vi "FourCC String to Int.vi"(10 "error in (no error)":errorcluster, 11 "fourCC String":string="MJPG") -> (2 "error out":errorcluster, 3 "fourCC Int":i32)   [LabVIEW 2014]
doc: "Help VI to convert the FourCC String to Int and back"
uses:
  Dependencies/x86/MSC I Process32.dll
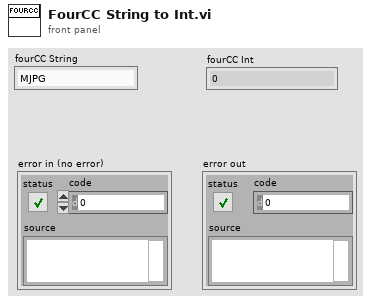
[diagram p1: front panel]
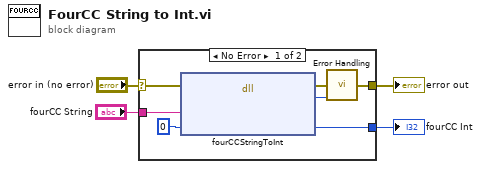
[diagram p0: block diagram]
diagram:
  n1 = case shown="No Error" "error in (no error)" {
    selector: "error in (no error)" -> [w9 w12]
    tunnel: [w8 w12] -> w4
    tunnel: "fourCC String" -> [w5 _]
    tunnel: [w6 _] -> w1
    frame No Error {
      n2 = dll-call lib="C:/Users/MSC/LabVIEW Projekte/LV 2014/MSC I-Process/user.lib/MSC-I Process/Dependencies/x86/MSC I Process*.dll" fn="fourCCStringToInt"(error in=w9, "fourCCString"=w5, "fourCCInt"=0) -> (error out=w11:errorcluster, "error"=w10:i32, "fourCCInt"=w6:i32)  [unwired: 3 in, 1 out]
      n3 = call "Error Handling.vi"("error in (no error)"=w11, "return type"=w10) -> ("error out"=w8:errorcluster)  [unwired: 12 in, 1 out]
    }
    frame Error {
    }
  }
  "error out" <- w4
  "fourCC Int" <- w1
